vi "Actor Core.vi"(8 "error in":errorcluster, 11 "Nested in":refnum<class "ButtonUI.lvclass">) -> (0 "error out":errorcluster, 3 "Actor out":refnum<class "Actor.lvclass">)   [LabVIEW 2021, in "ButtonUI.lvclass"]
doc: "(<B>Filename</B>: Actor Framework.lvlib:Actor.lvclass:Actor Core.vi)\n\nReceives messages to the actor, reacts to them, and initiates any error handling that may shut the actor down.\n\nDescendant classes may override this VI to append parallel tasks for the actor to complete while it handles messages. Overrides use the Call Parent Method node."
uses:
  ButtonUI.lvclass
  C:/Program Files (x86)/National Instruments/LabVIEW 2021/user.lib/John_Lib/AbstractActorTemplate/AbstractActorTemplate/UIActorTop.lvclass
  C:/Program Files (x86)/National Instruments/LabVIEW 2021/vi.lib/ActorFramework/Actor/Actor.lvclass
  <vilib>/ActorFramework/Actor/Actor.lvclass
  TopRef.ctl
  ButtonUI.lvclass/ButtonUI.ctl
  <vilib>/ActorFramework/Actor/Actor.lvclass/Actor.ctl
  <vilib>/ActorFramework/Message Enqueuer/Message Enqueuer.lvclass/Message Enqueuer.ctl
  <vilib>/ActorFramework/Message Enqueuer/Init from Existing Queue.vi
  <vilib>/ActorFramework/Message Enqueuer/Enqueue.vi
  <vilib>/ActorFramework/Stop Msg/Stop Msg.lvclass
  C:/Program Files (x86)/National Instruments/LabVIEW 2021/vi.lib/ActorFramework/Message/Message.lvclass
  <vilib>/ActorFramework/Message Priority Queue/Priority Enqueue.vi
  <vilib>/ActorFramework/Message Enqueuer/Message Enqueuer.lvclass
  <userlib>/John_Lib/AbstractActorTemplate/AbstractActorTemplate/UIActorTop.lvclass
  Button.ctl
panel:
  in  "MianTab_ButtonChoose":T1 caption="Radio Buttons"
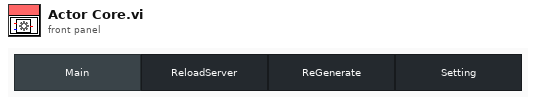
[diagram p1: front panel]
types:
  T1 = typedef "ButtonUI.lvclass/Button.ctl" = enum32{"Main", "Reload", "ReGenerate", "Setting"}
  T2 = typedef "ButtonUI.lvclass/TopRef.ctl" = cluster{"Str Refnum":refnum<vi>}
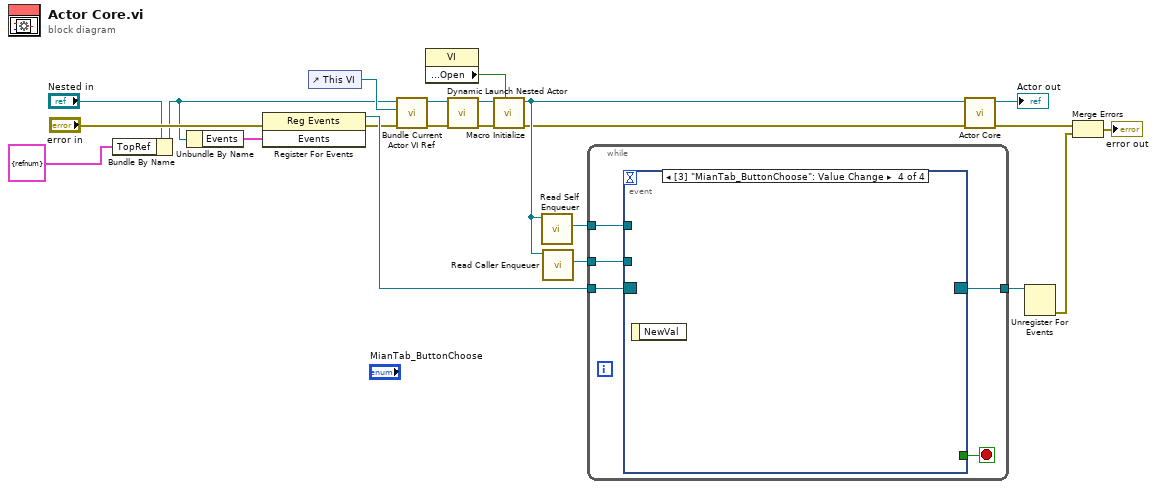
[diagram p0: block diagram]
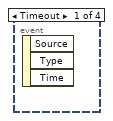
[diagram p2: hidden frame]
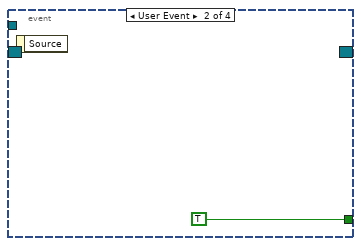
[diagram p3: hidden frame]
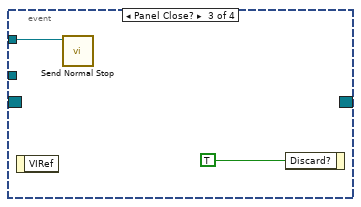
[diagram p4: hidden frame]
diagram:
  n1 = Bundle By Name(cluster="Nested in", "TopRef"=T2 {"Str Refnum"=refnum}) -> (w2:refnum<class "ButtonUI.lvclass">)
  n2 = Unbundle By Name(w2) -> ("Events"=w20:cluster{"Stop":refnum<user-event>})
  n3 = register-events ("Main Register for Events")(error in="error in", w20) -> (reference out=w21:refnum<event-registration>, error out=w5:errorcluster)  [unwired: 1 in]
  n4 = control-ref of="This VI"() -> (w3:refnum<vi>)
  n5 = call <userlib>:"Bundle Current Actor VI Ref.vi"("error in (no error)"=w5, "This VI"=w3, "UI ActorTop in"=w2) -> ("error out"=w4:errorcluster, "UI ActorTop out"=w6:refnum<class "ButtonUI.lvclass">)  [unwired: 6 in, 1 out]
  n6 = property class="VI"() -> ("Front Panel.Open"=w15:bool)  [unwired: 2 in, 2 out]
  n7 = call-dynamic "Dynamic Launch Nested Actor.vi"("error in (no error)"=w4, "UI ActorTop in"=w6) -> ("error out"=w16:errorcluster, "UI ActorTop out"=w17:refnum<class "ButtonUI.lvclass">)  [unwired: 8 in]
  n8 = call-dynamic "Macro Initialize.vi"("Front Panel Window:Open"=w15, "error in (no error)"=w16, "UI ActorTop in"=w17) -> ("error out"=w9:errorcluster, "UI ActorTop out"=w13:refnum<class "ButtonUI.lvclass">)  [unwired: 7 in]
  n9 = call <vilib>:"Read Self Enqueuer.vi"("Actor"=w13) -> ("Self Enqueuer"=w18:refnum<class "Message Enqueuer.lvclass">)  [unwired: 10 in]
  n10 = call <vilib>:"Read Caller Enqueuer.vi"("Actor"=w13) -> ("Caller Enqueuer"=w8:refnum<class "Message Enqueuer.lvclass">)  [unwired: 10 in]
  n11 = while {
    tunnel: w21 -> [w27]
    tunnel: [w25] -> w19
    tunnel: w18 -> [w24]
    tunnel: w8 -> [w23]
    stop <- w26 stop-if-true
    n12 = event "UI Events" shown="[3] \"MianTab_ButtonChoose\": Value Change" {
      selector: w27 -> [_ _ _ _]
      dyn-events: [_ _ _ _] -> w25
      timeout: _ -> [_ _ _ _]
      tunnel: [_ TRUE _ _] -> w26
      tunnel: w24 -> [_ _ w29 _]
      tunnel: w23 -> [_ _ _ _]
      event Timeout {
        n13 = event-data() -> ()  [unwired: 1 in, 3 out]
      }
      event User Event {
        n14 = event-data() -> ()  [unwired: 1 in, 1 out]
      }
      event Panel Close? {
        n15 = event-data() -> ()  [unwired: 1 in, 1 out]
        n16 = call <vilib>:"Send Normal Stop.vi"("Message Enqueuer"=w29) -> ()  [unwired: 10 in, 1 out]
        n17 = event-data("Discard?"=TRUE) -> ()  [unwired: 1 in, 1 out]
      }
      event Value Change {
        n18 = event-data() -> ()  [unwired: 1 in, 1 out]
      }
    }
  }
  n19 = call-parent "Actor Core.vi"("error in"=w9, "Actor in"=w13) -> ("error out"=w11:errorcluster, "Actor out"=→"Actor out":refnum<class "Actor.lvclass">)  [unwired: 8 in]
  n20 = Unregister For Events(event registration refnum=w19) -> (error out=w12:errorcluster)  [unwired: 1 in]
  n21 = Merge Errors(w11, w12) -> (→"error out":errorcluster)
